vi "light-sensor-indoor.vi"(7 "LabVIEW Web Service Request":refnum<class "Web Request.lvclass">) -> (2 "is-light-on":bool, 3 "light-gain-indoor":dbl)   [LabVIEW 2023]
uses:
  Sensors.vi
  PinoutSettings.vi
  <vilib>/wsapi/Web Request.lvclass
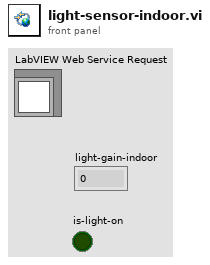
[diagram p1: front panel]
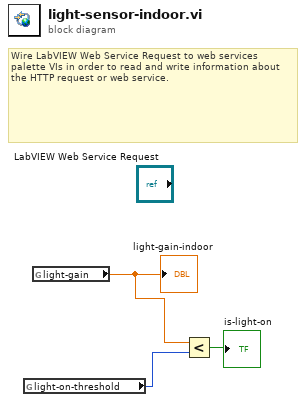
[diagram p0: block diagram]
diagram:
  # "Wire LabVIEW Web Service Request to web services palette VIs in order to read and write information about the HTTP request or web service."
  n1 = global read "PinoutSettings.vi" "light-on-threshold"() -> (w2:u8)
  n2 = global read "Sensors.vi" "light-gain"() -> (w3:dbl)
  "light-gain-indoor" <- w3
  n3 = Less?(x=w3, y=w2) -> (x < y?=→"is-light-on":bool)
